vi "NI 9237_Config.vi"(8 "error in":errorcluster, 11 "task in":refnum<k21>) -> (0 "error out":errorcluster, 3 "task out":refnum<k21>)   [LabVIEW 2025]
uses:
  <vilib>/DAQmx/create/channels.llb/DAQmx Create Channel (AI-Force-Bridge-Two-Point-Linear).vi
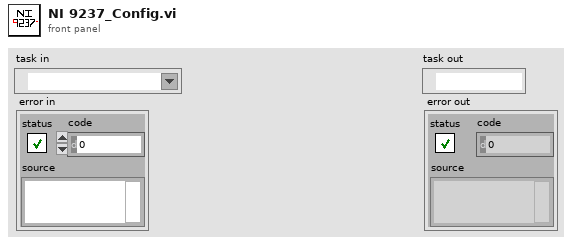
[diagram p1: front panel]
types:
  T1 = cluster{"bridge configuration":i32, "voltage excitation source":i32, "voltage excitation value":dbl, "nominal bridge resistance":dbl}
  T2 = cluster{"first electrical value":dbl, "second electrical value":dbl, "electrical units":i32, "first physical value":dbl, "second physical value":dbl, "physical units":i32}
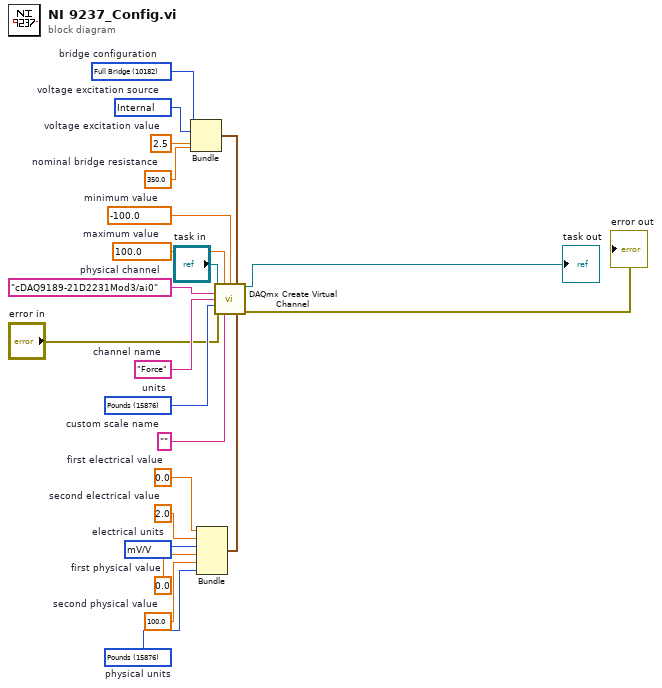
[diagram p0: block diagram]
diagram:
  w5 = 15876 items=["Newtons"=15875, "Pounds"=15876, "kgf"=15877]  # physical units
  w11 = 0.0  # first electrical value
  w10 = 2.0  # second electrical value
  w9 = 15897 items=["V/V"=15896, "mV/V"=15897]  # electrical units
  w8 = 0.0  # first physical value
  w7 = 100.0  # second physical value
  w13 = 350.0  # nominal bridge resistance
  w14 = 2.5  # voltage excitation value
  w15 = 10200 items=["Internal"=10200, "External"=10167]  # voltage excitation source
  w16 = 10182 items=["Full Bridge"=10182, "Half Bridge"=10187, "Quarter Bridge"=10270]  # bridge configuration
  w17 = 15876 items=["Newtons"=15875, "Pounds"=15876, "kgf"=15877, "From Custom Scale"=10065]  # units
  w18 = "Force"  # channel name
  w19 = ""  # custom scale name
  w20 = -100.0  # minimum value
  w21 = 100.0  # maximum value
  w22 = "cDAQ9189-21D2231Mod3/ai0"  # physical channel
  n1 = Bundle("bridge configuration"=w16, "voltage excitation source"=w15, "voltage excitation value"=w14, "nominal bridge resistance"=w13) -> (w12:T1)  [unwired: 1 in]
  n2 = Bundle("first electrical value"=w11, "second electrical value"=w10, "electrical units"=w9, "first physical value"=w8, "second physical value"=w7, "physical units"=w5) -> (w6:T2)  [unwired: 1 in]
  n3 = call-poly <vilib>:"DAQmx Create Virtual Channel.vi"("task in"="task in", "maximum value"=w21, "minimum value"=w20, "bridge information"=w12, "physical channels"=w22, "name to assign"=w18, "units"=w17, "error in"="error in", "custom scale name"=w19, "scaling information"=w6) -> ("task out"=→"task out":refnum<k21>, "error out"=→"error out":errorcluster)  [unwired: 4 in]
